vi "Make from Test Case Path.vi"(8 "error in (no error)":errorcluster, 10 "Test Case":path) -> (0 "error out":errorcluster, 3 "LUnit Test Suite V2 out":refnum<class "LUnit Test Suite V2.lvclass">)   [LabVIEW 2020, in "LUnit Test Suite V2.lvclass"]
uses:
  LUnit Test Suite V2.lvclass
  Result/Type.ctl
  LUnit Test Suite V2.lvclass/LUnit Test Suite V2.ctl
  LUnit Test Case/LUnit Test Case V2.lvclass
  C:/Git/astemes-lunit/source/Rewrite Project/Run/Runnable.lvclass
  Result/Result.lvlib
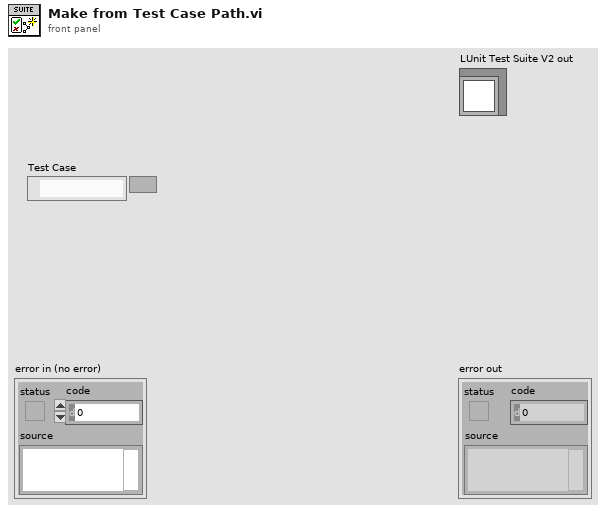
[diagram p1: front panel]
types:
  T1 = typedef "Result.lvlib/Type.ctl" = enum16{"Method", "Case", "Suite", "Pass", "Fail", "Skip", "Pass if", "Fail if", "Pass if Error", "Fail if Error", "Pass if Equal", "Fail if Equal"}
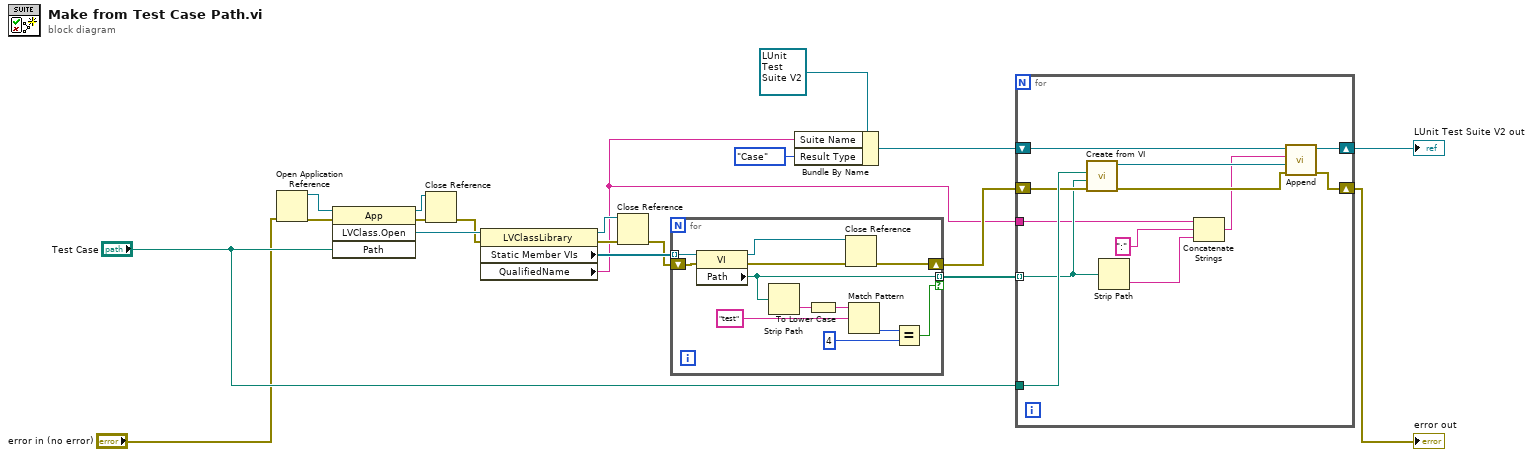
[diagram p0: block diagram]
diagram:
  n1 = Open Application Reference(8:"error in (no error)") -> (0:w17:errorcluster, 3:w18:refnum<vi>)  [unwired: 3 in]
  n2 = invoke class="App" method="LVClass.Open"(reference=w18, error in=w17, "Path"="Test Case") -> (reference out=w4:refnum<vi>, error out=w15:errorcluster, "LVClass.Open"=w16:refnum<vi>)  [unwired: 1 in, 1 out]
  n3 = Close Reference(reference=w4, error in (no error)=w15) -> (error out=w5:errorcluster)
  n4 = property class="LVClassLibrary"(reference=w16, error in=w5) -> (reference out=w6:refnum<vi>, error out=w9:errorcluster, "Static Member VIs"=w14:refnum<vi>[], "QualifiedName"=w1:string)
  n5 = Close Reference(reference=w6, error in (no error)=w9) -> (error out=w7:errorcluster)
  n6 = for {
    tunnel: w14 -> [w32] mode=indexing
    tunnel: [w22] -> w13 mode=indexing if=w27
    shift-right: [w24] -> w8
    shift-left: w7 -> [w26]
    n7 = property class="VI"(reference=w32, error in=w26) -> (reference out=w23:refnum<vi>, error out=w25:errorcluster, "Path"=w22:path)
    n8 = Strip Path(path=w22) -> (name=w21:string)  [unwired: 1 out]
    n9 = To Lower Case(string=w21) -> (all lower case string=w30:string)
    n10 = Close Reference(reference=w23, error in (no error)=w25) -> (error out=w24:errorcluster)
    n11 = Match Pattern(string=w30, regular expression="test") -> (offset past match=w29:i32)  [unwired: 1 in, 3 out]
    n12 = Equal?(x=w29, y=4) -> (x = y?=w27:bool)
  }
  n13 = Bundle By Name(cluster=refnum<class "LUnit Test Suite V2.lvclass"> refnum ("LUnit Test Suite V2 in"), "Suite Name"=w1, "Result Type"=Type."Case") -> (w3:refnum<class "LUnit Test Suite V2.lvclass">)
  n14 = for {
    tunnel: "Test Case" -> [w44]
    tunnel: w13 -> [w37] mode=indexing
    shift-right: [w42] -> w11
    shift-left: w3 -> [w43]
    shift-right: [w40] -> w10
    shift-left: w8 -> [w39]
    tunnel: w1 -> [w34]
    n15 = call "Create from VI.vi"("error in (no error)"=w39, "Test Method VI Path"=w37, "Test Case LVCLass Path"=w44) -> ("error out"=w41:errorcluster, "LUnit Test Case V2 out"=w38:refnum<class "LUnit Test Case V2.lvclass">)  [unwired: 7 in]
    n16 = Strip Path(path=w37) -> (name=w35:string)  [unwired: 1 out]
    n17 = Concatenate Strings(w34, ":" ("string"), w35) -> (w33:string)
    n18 = call "Append.vi"("error in (no error)"=w41, "Runnable"=w38, "Name"=w33, "LUnit Test Suite V2 in"=w43) -> ("error out"=w40:errorcluster, "LUnit Test Suite V2 out"=w42:refnum<class "LUnit Test Suite V2.lvclass">)  [unwired: 6 in]
  }
  "error out" <- w10
  "LUnit Test Suite V2 out" <- w11
